vi "AlliGator Get I-m-phi Dataset Phasor Harmonic Components.vi"(8 "Error In":errorcluster, 11 "Harmonic Data":T1[](array[typedef])) -> (0 "Error Out":errorcluster, 1 "Harmonic Order":u8[](array[numeric]), 3 "Phasor Components":sgl[][][](array[numeric]))   [LabVIEW 2021, in "AlliGator Files.lvlib"]
doc: "Converts FLIMBox data structure to one used internally in AlliGator."
uses:
  AlliGator Files.lvlib
  FLIMbox/FLIMbox Harmonic Data.ctl
  FLIMbox/FLIMBox.lvlib
panel:
  # "see the AlliGator License on the block diagram (Ctrl+E or Window:Show Block Diagram)"
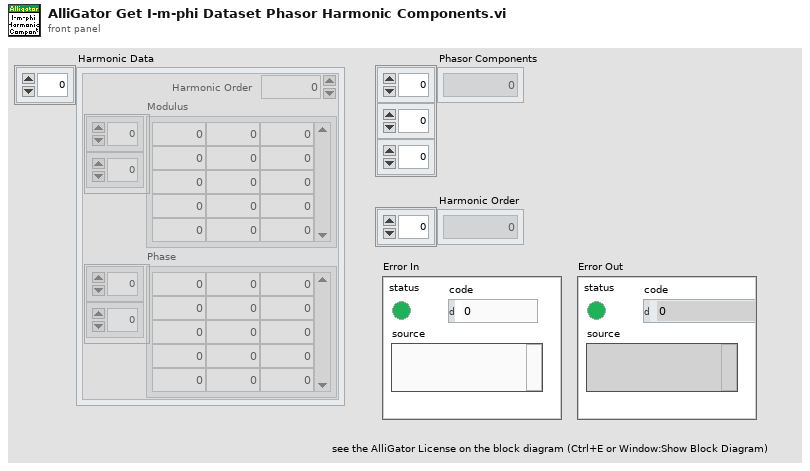
[diagram p1: front panel]
types:
  T1 = typedef "FLIMBox.lvlib/FLIMbox Harmonic Data.ctl" = cluster{"Modulus":sgl[][], "Phase":sgl[][], "Harmonic Order":u8}
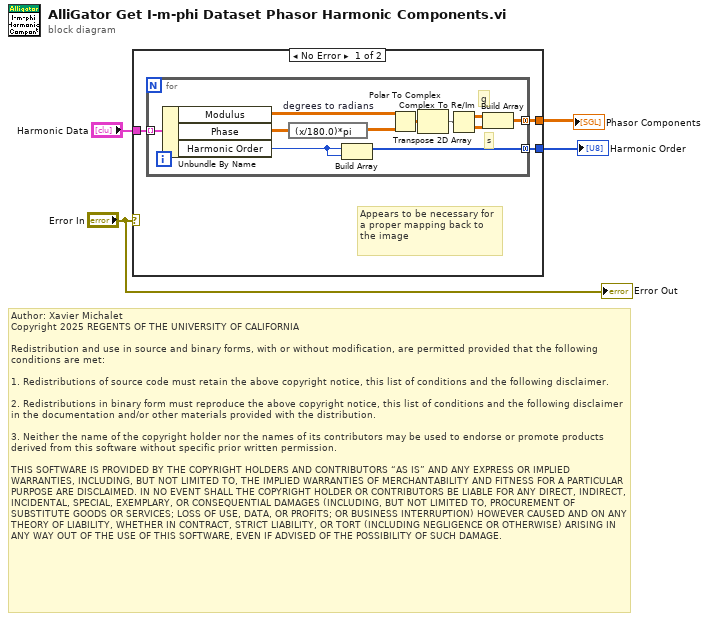
[diagram p0: block diagram]
diagram:
  # "Author: Xavier Michalet\nCopyright 2025 REGENTS OF THE UNIVERSITY OF CALIFORNIA\n\nRedistribution and use in source and binary forms, with or without modification, are permitted provided that the following conditions are met:\n\n1. Redistributions of source code must retain the above copyright notice, this list of conditions and the following disclaimer.\n\n2. Redistributions in binary form must reproduce the above copyright notice, this list of conditions and the following disclaimer in the documentation and/or other materials provided with the distribution.\n\n3. Neither the name of the copyright holder nor the names of its contributors may be used to endorse or promote products derived from this software without specific prior written permission.\n\nTHIS SOFTWARE IS PROVIDED BY THE COPYRIGHT HOLDERS AND CONTRIBUTORS “AS IS” AND ANY EXPRESS OR IMPLIED WARRANTIES, INCLUDING, BUT NOT LIMITED TO, THE IMPLIED WARRANTIES OF MERCHANTABILITY AND FITNESS FOR A PARTICULAR PURPOSE ARE DISCLAIMED. IN NO EVENT SHALL THE COPYRIGHT HOLDER OR CONTRIBUTORS BE LIABLE FOR ANY DIRECT, INDIRECT, INCIDENTAL, SPECIAL, EXEMPLARY, OR CONSEQUENTIAL DAMAGES (INCLUDING, BUT NOT LIMITED TO, PROCUREMENT OF SUBSTITUTE GOODS OR SERVICES; LOSS OF USE, DATA, OR PROFITS; OR BUSINESS INTERRUPTION) HOWEVER CAUSED AND ON ANY THEORY OF LIABILITY, WHETHER IN CONTRACT, STRICT LIABILITY, OR TORT (INCLUDING NEGLIGENCE OR OTHERWISE) ARISING IN ANY WAY OUT OF THE USE OF THIS SOFTWARE, EVEN IF ADVISED OF THE POSSIBILITY OF SUCH DAMAGE."
  n1 = case shown="No Error" "Error In" {
    tunnel: "Harmonic Data" -> [w7 _]
    tunnel: [w6 _] -> w3
    tunnel: [w5 _] -> w1
    frame No Error {
      # "Appears to be necessary for a proper mapping back to  the image"
      n2 = for {
        tunnel: w7 -> [w18] mode=indexing
        tunnel: [w16] -> w6 mode=concatenating
        tunnel: [w10] -> w5 mode=concatenating
        # "s"
        # "g"
        n3 = Unbundle By Name(w18) -> ("Modulus"=w13:sgl[][], "Phase"=w15:sgl[][], "Harmonic Order"=w17:u8)
        n4 = expression code="(x/180.0)*pi" "degrees to radians"(w15) -> (w14:sgl[][])
        n5 = Build Array(w17, w17) -> (w16:u8[])
        n6 = Polar To Complex(1:w14, 2:w13) -> (0:w12:csg[][])
        n7 = Transpose 2D Array(2D array=w12) -> (transposed array=w8:csg[][])
        n8 = Complex To Re/Im(x + iy=w8) -> (x=w11:sgl[][], y=w9:sgl[][])
        n9 = Build Array(w11, w9) -> (w10:sgl[][][])
      }
    }
    frame Error {
    }
  }
  "Harmonic Order" <- w3
  "Phasor Components" <- w1
  "Error Out" <- "Error In"
